vi "List Stream Buffer Contents.vi"(8 "error in (no error)":errorcluster, 9 "Device Number":string, 10 "Buffer Number (1)":i32=1, 11 "VISA resource name":refnum<visa-resource-name>) -> (0 "error out":errorcluster, 2 "Buffer Contents":string[](array[string]), 3 "VISA resource name out":refnum<visa-resource-name>)   [LabVIEW 2015, in "Zaber A Series.lvlib"]
doc: "Lists all of the commands currently stored in the specified stream buffer. The input must be a number between 1 and the value of the \"stream.numbufs\" device setting, which can be retrieved with the Get Stream Support Info VI. Zero is not a valid input; live stream contents cannot be listed because they are continually consumed. The output is an array of strings, one command per entry. Output is empty in the case of an error.\n\nThis VI does not check in advance for error conditions such as streams not being supported.\n\nThis VI requires that the Initialize VI has been called with the same serial port."
uses:
  Zaber A Series.lvlib
  Private/All Commands.ctl
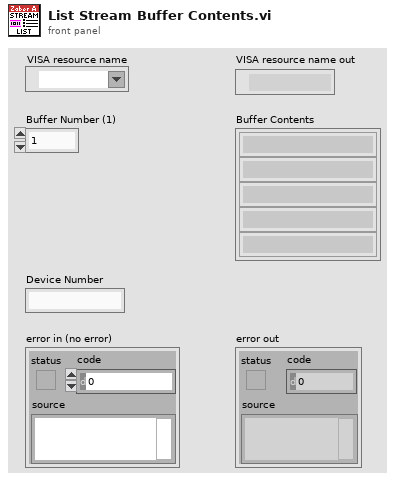
[diagram p1: front panel]
types:
  T1 = typedef "Zaber A Series.lvlib/All Commands.ctl" = string
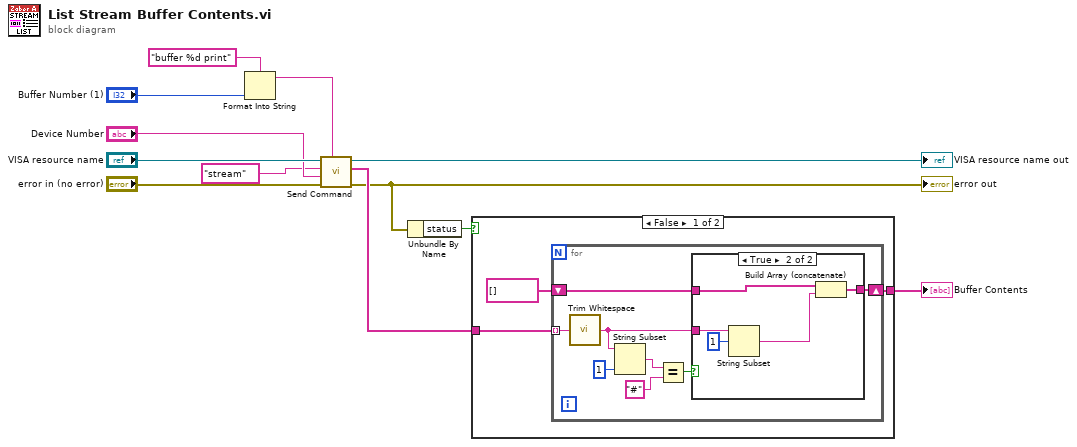
[diagram p0: block diagram]
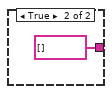
[diagram p3: hidden frame]
diagram:
  n1 = Format Into String(format string="buffer %d print", "Buffer Number (1)") -> (resulting string=w4:string)  [unwired: 2 in, 1 out]
  n2 = call "Send Command.vi"("Data"=w4, "error in (no error)"="error in (no error)", "Device and Axis"="Device Number", "Command"=T1 "stream" ("Complete Command List"), "VISA resource name"="VISA resource name") -> ("error out"=w2:errorcluster, "Response String Array"=w8:string[], "VISA resource name out"=→"VISA resource name out":refnum<visa-resource-name>)  [unwired: 1 in, 3 out]
  "error out" <- w2
  n3 = Unbundle By Name(w2) -> ("status"=w9:bool)
  n4 = case shown="False" w9 {
    tunnel: w8 -> [w15 _]
    tunnel: [w14 string[] []] -> w7
    frame False {
      n5 = for {
        tunnel: w15 -> [w23] mode=indexing
        shift-right: [w17] -> w14
        shift-left: string[] [] -> [w16]
        n6 = call <vilib>:"Trim Whitespace.vi"("string"=w23) -> ("trimmed string"=w18:string)  [unwired: 1 in]
        n7 = String Subset(string=w18, length (rest)=1 ("length (rest)")) -> (substring=w21:string)  [unwired: 1 in]
        n8 = Equal?(x=w21, y="#") -> (x = y?=w19:bool)
        n9 = case shown="True" w19 {
          tunnel: w18 -> [_ w27]
          tunnel: [w24 w29] -> w17
          tunnel: w16 -> [w24 w28]
          frame False {
          }
          frame True {
            n10 = String Subset(string=w27, offset (0)=1) -> (substring=w25:string)  [unwired: 1 in]
            n11 = Build Array (concatenate)(w28, w25) -> (w29:string[])
          }
        }
      }
    }
    frame True {
    }
  }
  "Buffer Contents" <- w7
